vi "Connect to Slave.vi"(8 "error in (no error)":errorcluster, 11 "TCP master in":refnum<class "SMSD Master.lvclass">) -> (0 "error out":errorcluster, 3 "TCP master out":refnum<class "SMSD Master.lvclass">)   [LabVIEW 2021, in "SMSD Master.lvclass"]
doc: "Opens a TCP connection to the address and port stored in the class."
uses:
  SMSD Master.lvclass
  SMSD Master.lvclass/SMSD Master.ctl
  Transmission Data Unit/SMSD/SMSD ADU.lvclass/SMSD ADU.ctl
  Modbus_v121c/Network Interface/TCP Interface/TCP Shared Components/TCP Read.vi
  Transmission Data Unit/SMSD/close connection.vi
  <vilib>/Utility/error.llb/Clear Errors.vi
  Transmission Data Unit/SMSD/SMSD ADU.lvclass
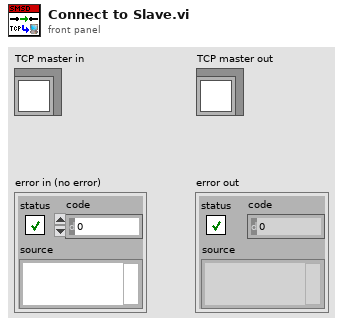
[diagram p1: front panel]
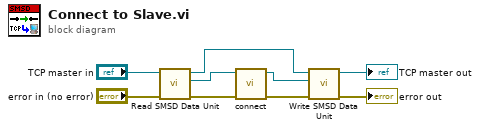
[diagram p0: block diagram]
diagram:
  n1 = call "Read SMSD Data Unit.vi"("error in (no error)"="error in (no error)", "SMSD Master in"="TCP master in") -> ("error out"=w4:errorcluster, "IP Data Unit"=w3:refnum<class "SMSD ADU.lvclass">, "SMSD Master out"=w9:refnum<class "SMSD Master.lvclass">)  [unwired: 7 in]
  n2 = call "connect.vi"("error in (no error)"=w4, "IP simple ADU in"=w3) -> ("error out"=w1:errorcluster, "IP simple ADU out"=w2:refnum<class "SMSD ADU.lvclass">)  [unwired: 8 in]
  n3 = call "Write SMSD Data Unit.vi"("error in (no error)"=w1, "IP Data Unit"=w2, "SMSD Master in"=w9) -> ("error out"=→"error out":errorcluster, "SMSD Master out"=→"TCP master out":refnum<class "SMSD Master.lvclass">)  [unwired: 7 in]
